vi "GPS HeadingChange Event Example.vi"() -> ()   [LabVIEW 2012, in "Phidget GPS.lvlib"]
uses:
  <instrlib>/Phidgets/Phidget GPS/Phidget GPS.lvlib
  <instrlib>/Phidgets/Phidget GPS/Public/GPSStart.vi
  <instrlib>/Phidgets/Phidget GPS/Public/GPSClose.vi
  <instrlib>/Phidgets/Phidget Common/Phidget Common.lvlib
panel:
  out "Heading":dbl caption="Longitude"
  out "Velocity":dbl caption="Altitude"
  in  "stop":bool
  out "Serial Number Return":i32
  in  "Device Info":T1={"Serial Number"=-1, "Channel"=0, "Port"=0}
  out "error out":errorcluster
  # "Be sure to use this stop button to stop the program.\nIf you use the \"Abort Execution\" button, you will\nneed to use PhidgetResetLibrary.vi or restart Labview \nin order for any Phidgets to work."
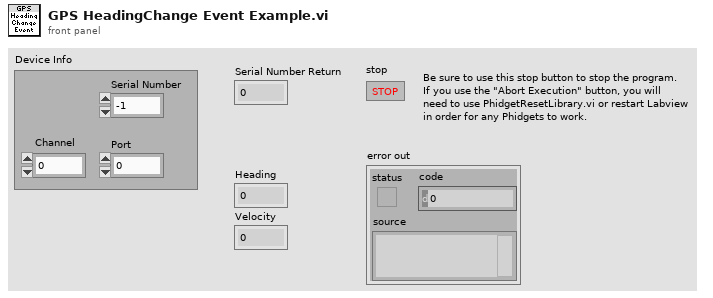
[diagram p1: front panel]
types:
  T1 = cluster{"Serial Number":i32, "Channel":i32, "Port":i32}
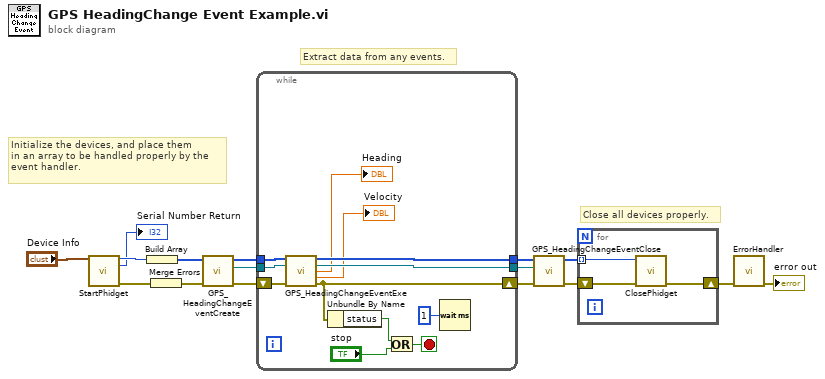
[diagram p0: block diagram]
diagram:
  # "Close all devices properly."
  # "Extract data from any events."
  # "Initialize the devices, and place them\nin an array to be handled properly by the\nevent handler."
  n1 = call-poly <instrlib>:"StartPhidget.vi"("Device Info"="Device Info") -> ("Phidget ID"=w5:u64, "Serial Number Return"=→"Serial Number Return":i32, "error out"=w1:errorcluster)  [unwired: 11 in, 1 out]
  n2 = Build Array(w5) -> (w16:u64[])
  n3 = Merge Errors(w1) -> (w7:errorcluster)
  n4 = call <instrlib>:"GPS_HeadingChangeEventCreate.vi"("error in (no error)"=w7, "Devices In"=w16) -> ("error out"=w9:errorcluster, "Event Registration Refnum"=w14:refnum<event-registration>, "Devices Out"=w15:u64[])  [unwired: 7 in]
  n5 = while {
    tunnel: w15 -> [w28]
    tunnel: w14 -> [w23]
    tunnel: [w27] -> w11
    shift-right: [w22] -> w10
    shift-left: w9 -> [w26]
    tunnel: [w24] -> w3
    stop <- w21 stop-if-true
    n6 = call <instrlib>:"GPS_HeadingChangeEventExe.vi"("Devices In"=w28, "Event Registration Refnum In"=w23, "error in (no error)"=w26) -> ("Devices Out"=w24:u64[], "Event Registration Refnum Out"=w27:refnum<event-registration>, "Heading"=→"Heading":dbl, "Velocity"=→"Velocity":dbl, "error out"=w22:errorcluster)  [unwired: 5 in, 3 out]
    n7 = Unbundle By Name(w22) -> ("status"=w19:bool)
    n8 = Or(x=w19, y="stop") -> (x .or. y?=w21:bool)
    n9 = Wait (ms)(milliseconds to wait=u32 1) -> ()  [unwired: 1 out]
  }
  n10 = call <instrlib>:"GPS_HeadingChangeEventClose.vi"("error in (no error)"=w10, "Event Registration Refnum In"=w11, "Devices In"=w3) -> ("error out"=w6:errorcluster, "Devices Out"=w4:u64[])  [unwired: 7 in]
  n11 = for {
    tunnel: w4 -> [w29] mode=indexing
    shift-right: [w31] -> w13
    shift-left: w6 -> [w30]
    n12 = call-poly <instrlib>:"ClosePhidget.vi"("error in"=w30, "Device In"=w29) -> ("error out"=w31:errorcluster)  [unwired: 9 in]
  }
  n13 = call <instrlib>:"ErrorHandler.vi"("error in"=w13) -> ("error out"=→"error out":errorcluster)  [unwired: 9 in, 1 out]
